vi "Digitizer Parse Channel String.vi"(0 "Channel List":string) -> (1 "Dig2 Channels":string, 2 "Dig2 Used?":bool, 3 "Dig1 Channels":string, 4 "Dig1 Used?":bool)   [LabVIEW 2010]
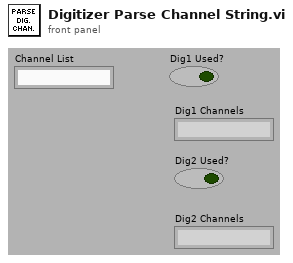
[diagram p1: front panel]
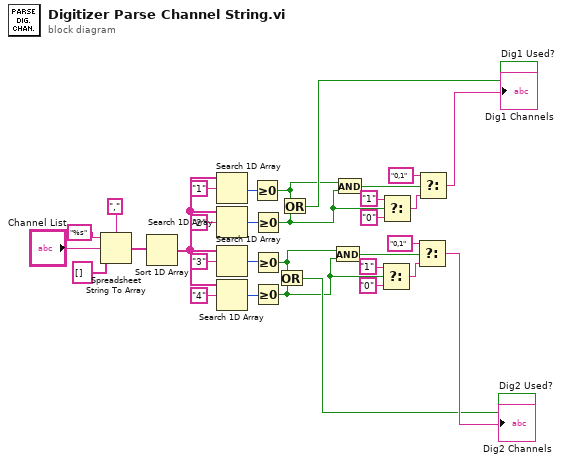
[diagram p0: block diagram]
diagram:
  n1 = Spreadsheet String To Array(delimiter (Tab)=",", format string="%s", spreadsheet string="Channel List", array type (2D Dbl)=string[] []) -> (array=w4:string[])
  n2 = Sort 1D Array(array=w4) -> (sorted array=w5:string[])
  n3 = Search 1D Array(1D array=w5, element="1") -> (index of element=w10:i32)  [unwired: 1 in]
  n4 = Search 1D Array(1D array=w5, element="2") -> (index of element=w13:i32)  [unwired: 1 in]
  n5 = Search 1D Array(1D array=w5, element="3") -> (index of element=w12:i32)  [unwired: 1 in]
  n6 = Search 1D Array(1D array=w5, element="4") -> (index of element=w11:i32)  [unwired: 1 in]
  n7 = Greater Or Equal To 0?(x=w10) -> (x >= 0?=w14:bool)
  n8 = Greater Or Equal To 0?(x=w13) -> (x >= 0?=w18:bool)
  n9 = Greater Or Equal To 0?(x=w12) -> (x >= 0?=w15:bool)
  n10 = Greater Or Equal To 0?(x=w11) -> (x >= 0?=w27:bool)
  n11 = Or(x=w15, y=w27) -> (x .or. y?=→"Dig2 Used?":bool)
  n12 = Or(x=w14, y=w18) -> (x .or. y?=→"Dig1 Used?":bool)
  n13 = And(x=w15, y=w27) -> (x .and. y?=w26:bool)
  n14 = And(x=w14, y=w18) -> (x .and. y?=w16:bool)
  n15 = Select(t="1", s=w27, f="0") -> (s? t:f=w24:string)
  n16 = Select(t="1", s=w18, f="0") -> (s? t:f=w20:string)
  n17 = Select(t="0,1", s=w26, f=w24) -> (s? t:f=→"Dig2 Channels":string)
  n18 = Select(t="0,1", s=w16, f=w20) -> (s? t:f=→"Dig1 Channels":string)
